vi "Launch Event Handler.vi"(8 "error in (no error)":errorcluster, 10 "EventAggregator In":refnum<class "IEventAggregator.lvclass">, 11 "EventHandler In":refnum<class "IEventHandler.lvclass">) -> (0 "error out":errorcluster, 1 "Registration Done Notifier":refnum<notifier>, 2 "EventAggregator Out":refnum<class "IEventAggregator.lvclass">, 3 "EventHandler Enqueuer":refnum<class "Message Enqueuer.lvclass">)   [LabVIEW 2017, in "ActorEvents.lvlib" / "IEventHandler.lvclass"]
uses:
  IEventHandler.lvclass
  C:/Program Files (x86)/National Instruments/LabVIEW 2017/vi.lib/ActorFramework/Actor/Actor.lvclass
  IEventAggregator/IEventAggregator.lvclass
  <vilib>/ActorFramework/Message Enqueuer/Message Enqueuer.lvclass
  <vilib>/ActorFramework/Actor/Actor.lvclass/Actor.ctl
  <vilib>/ActorFramework/Message Enqueuer/Message Enqueuer.lvclass/Message Enqueuer.ctl
  IEventHandler.lvclass/IEventHandler.ctl
  <vilib>/ActorFramework/Message Enqueuer/Init from Existing Queue.vi
  <vilib>/ActorFramework/Actor/Actor.lvclass
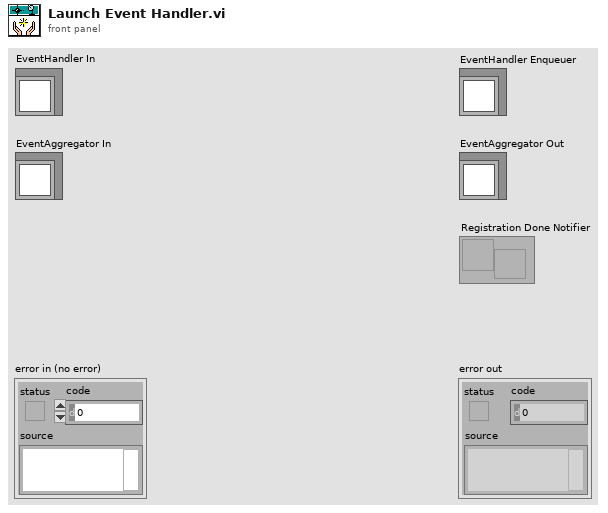
[diagram p1: front panel]
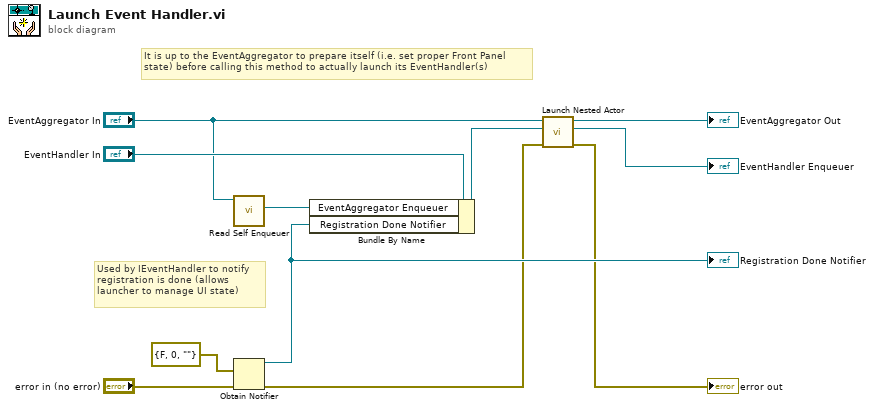
[diagram p0: block diagram]
diagram:
  # "Used by IEventHandler to notify\nregistration is done (allows\nlauncher to manage UI state)"
  # "It is up to the EventAggregator to prepare itself (i.e. set proper Front Panel\nstate) before calling this method to actually launch its EventHandler(s)"
  n1 = call <vilib>:"Read Self Enqueuer.vi"("Actor"="EventAggregator In") -> ("Self Enqueuer"=w3:refnum<class "Message Enqueuer.lvclass">)  [unwired: 10 in]
  n2 = Obtain Notifier(notification data type=errorcluster {"status"=FALSE, "code"=0, "source"=""} ("error constant"), error in (no error)="error in (no error)") -> (notifier out=w11:refnum<notifier>, error out=w1:errorcluster)  [unwired: 2 in, 1 out]
  "Registration Done Notifier" <- w11
  n3 = Bundle By Name(cluster="EventHandler In", "EventAggregator Enqueuer"=w3, "Registration Done Notifier"=w11) -> (w7:refnum<class "IEventHandler.lvclass">)
  n4 = call <vilib>:"Launch Nested Actor.vi"("error in (no error)"=w1, "Nested Actor"=w7, "Caller Actor in"="EventAggregator In") -> ("error out"=→"error out":errorcluster, "Nested Actor's Enqueuer"=→"EventHandler Enqueuer":refnum<class "Message Enqueuer.lvclass">, "Caller Actor out"=→"EventAggregator Out":refnum<class "IEventAggregator.lvclass">)  [unwired: 6 in]
